vi "Launch DAQ Actor.vi"(8 "error in (no error)":errorcluster, 10 "AI Driver":refnum<class "AI Driver.lvclass">[](array[class]), 11 "DAQ Controller":refnum<class "DAQ Controller.lvclass">) -> (0 "error out":errorcluster, 3 "DAQ Controller":refnum<class "DAQ Controller.lvclass">)   [LabVIEW 2022 SP3, in "DAQ Process.lvlib" / "DAQ Process.lvclass"]
uses:
  DAQ Process.lvclass
  AI Driver/AI Driver.lvclass
  DAQ Controller/DAQ Controller.lvclass
  C:/Program Files/National Instruments/LabVIEW 2022/vi.lib/ActorFramework/Actor/Actor.lvclass
  DAQ Process.lvclass/DAQ Process.ctl
  <vilib>/ActorFramework/Actor/Actor.lvclass
  XY Stage/Process Actor/Process Framework/Process State Data/Process State Data.lvclass
  XY Stage/Process Actor/Process Framework/Interlock Q Class/Interlock Q Class.lvclass
  DAQ Data/DAQ Data.lvclass
  C:/Program Files/National Instruments/LabVIEW 2022/vi.lib/MGI/Monitored Actor/Monitored Actor/Monitored Actor/Monitored Actor.lvclass
  C:/XY Stage/IO Monitor/DAQ Actor/DAQ Actor/DAQ Process.lvclass
  C:/XY Stage/IO Monitor/Aquire Data/Aquire Data.lvclass
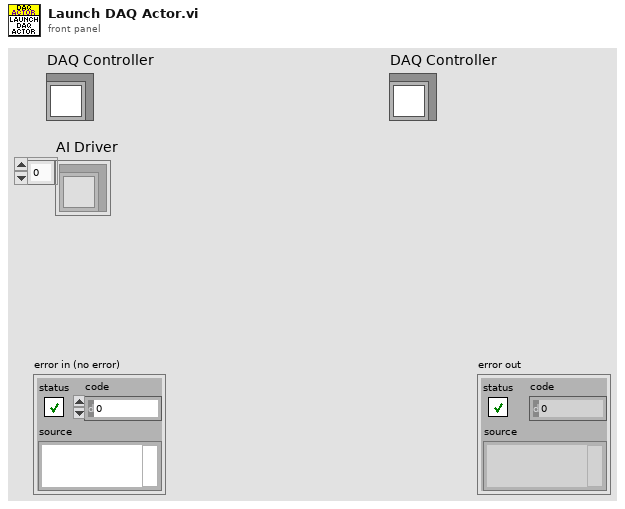
[diagram p1: front panel]
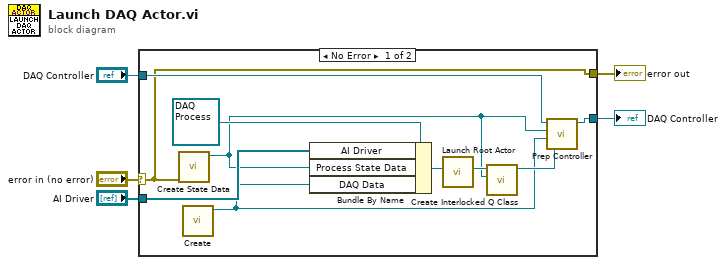
[diagram p0: block diagram]
diagram:
  n1 = case shown="No Error" "error in (no error)" {
    selector: "error in (no error)" -> [w7 w17]
    tunnel: [w7 w17] -> w4
    tunnel: "AI Driver" -> [w13 _]
    tunnel: "DAQ Controller" -> [w11 w16]
    tunnel: [w10 w16] -> w1
    frame No Error {
      n2 = call "Create State Data.vi"("error in (no error)"=w7) -> ("Process State Data out"=w8:refnum<data-value>)  [unwired: 9 in, 1 out]
      n3 = call "Create.vi"() -> ("DAQ Data"=w6:refnum<data-value>)  [unwired: 10 in, 1 out]
      n4 = Bundle By Name(cluster=refnum<class "DAQ Process.lvclass"> refnum ("DAQ Actor.lvlib:DAQ Actor.lvclass"), "AI Driver"=w13, "Process State Data"=w8, "DAQ Data"=w6) -> (w14:refnum<class "DAQ Process.lvclass">)
      n5 = call <vilib>:"Launch Root Actor.vi"("Actor"=w14) -> ("Actor's Enqueuer"=w12:refnum<class "Message Enqueuer.lvclass">)  [unwired: 9 in, 1 out]
      n6 = call "Create Interlocked Q Class.vi"("Process State Data"=w8, "Process Q"=w12) -> ("Interlock Q Class out"=w9:refnum<class "Interlock Q Class.lvclass">)  [unwired: 9 in]
      n7 = call "Prep Controller.vi"("Interlock Q Class"=w9, "DAQ Data"=w6, "Process State Data"=w8, "DAQ Controller in"=w11) -> ("DAQ Controller out"=w10:refnum<class "DAQ Controller.lvclass">)  [unwired: 6 in, 1 out]
    }
    frame Error {
    }
  }
  "error out" <- w4
  "DAQ Controller" <- w1
